vi "LVClass_CameraSet dtor.vi"(0 "CameraSet.lvclass":refnum<class "CameraSet.lvclass">, 11 "error in (no error)":errorcluster) -> (4 "CameraSet.lvclass":refnum<class "CameraSet.lvclass">, 15 "error out":errorcluster)   [LabVIEW 2020, in "CameraSet.lvclass"]
doc: "CameraSet destructor.\n\n--------------------------------------------------------------------------------\n\n<B>camera_setIn </B> : CameraSet object.\n<B>camera_setOut </B> : CameraSet object.\n<B>ErrorIn </B> : Error\n<B>ErrorOut </B> : Error\n\n--------------------------------------------------------------------------------"
uses:
  CameraSet.lvclass
  CameraSet.lvclass/CameraSet.ctl
  CameraSet.ctl
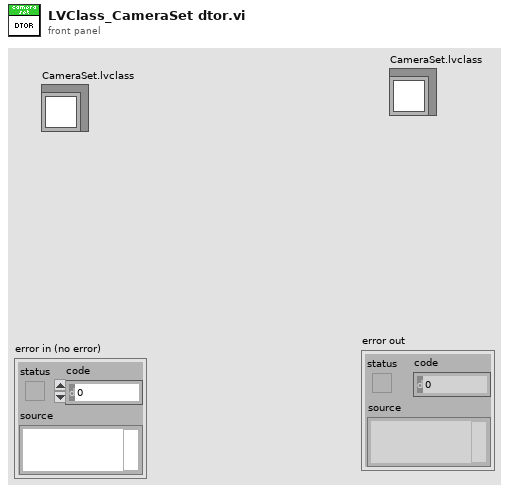
[diagram p1: front panel]
types:
  T1 = typedef "CameraSet.ctl" = i32
  T2 = typedef "Handle creation.ctl" = enum16{"By ctor", "By write function"}
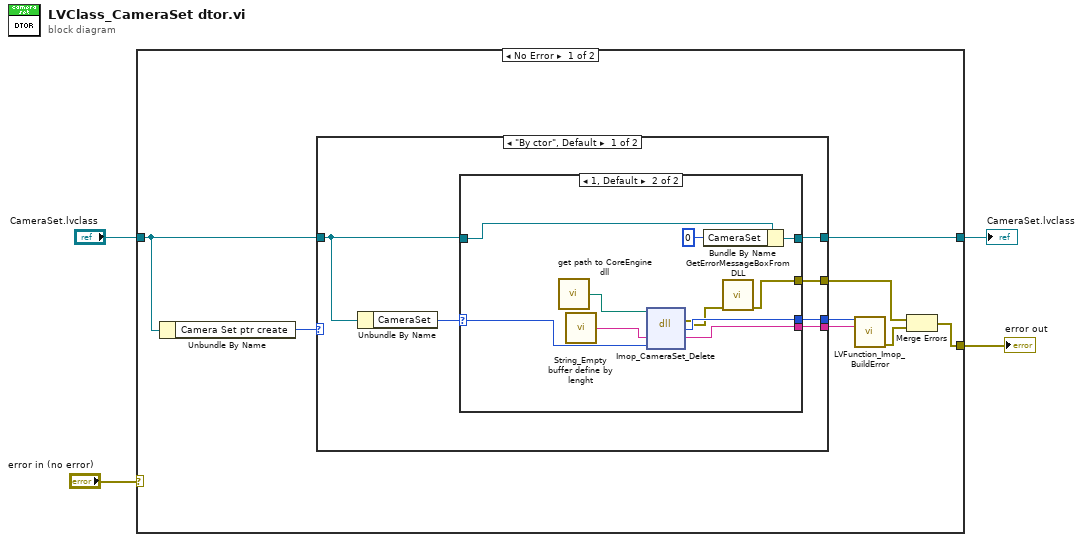
[diagram p0: block diagram]
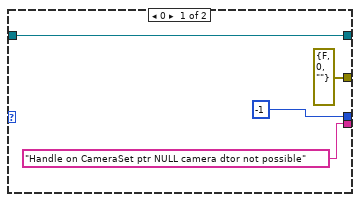
[diagram p2: hidden frame]
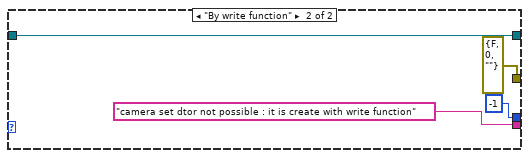
[diagram p3: hidden frame]
diagram:
  n1 = case shown="No Error" "error in (no error)" {
    selector: "error in (no error)" -> [_ w37]
    tunnel: "CameraSet.lvclass" -> [w9 w38]
    tunnel: [w10 w38] -> w2
    tunnel: [w5 w37] -> w1
    frame No Error {
      n2 = Unbundle By Name(w9) -> ("Camera Set ptr create"=w8:T2)
      n3 = case shown="\"By ctor\", Default" w8 {
        tunnel: [w18 "camera set dtor not possible : it is create with write function" ("message")] -> w12
        tunnel: [w17 -1] -> w11
        tunnel: [w16 w34] -> w10
        tunnel: w9 -> [w15 w34]
        tunnel: [w13 errorcluster {"status"=FALSE, "code"=0, "source"=""} ("error OUT")] -> w7
        frame "By ctor", Default {
          n4 = Unbundle By Name(w15) -> ("CameraSet"=w14:T1)
          n5 = case shown="1, Default" w14 {
            selector: w14 -> [_ w29]
            tunnel: ["Handle on CameraSet ptr NULL camera dtor not possible" ("message") w31] -> w18
            tunnel: [-1 w30] -> w17
            tunnel: w15 -> [w20 w26]
            tunnel: [w20 w25] -> w16
            tunnel: [errorcluster {"status"=FALSE, "code"=0, "source"=""} ("error OUT") w23] -> w13
            frame 0 {
            }
            frame 1, Default {
              n6 = call "get path to CoreEngine dll.vi"() -> ("path to c_interface_vc100.dll"=w28:path)  [unwired: 12 in, 3 out]
              n7 = call "String_Empty buffer define by lenght.vi"() -> ("Empty buffer"=w32:string)  [unwired: 1 in]
              n8 = dll-call lib="D:/soft/HASO_v3/SVN_trunk/ImOpCoreEngine4_LV2011/DLLs/c_interface_vc100.dll" fn="Imop_CameraSet_Delete"(path in=w28, "message"=w32, "objet"=w29) -> (error out=w27:errorcluster, "return type"=w30:i32, "message"=w31:string)  [unwired: 3 in, 1 out]
              n9 = Bundle By Name(cluster=w26, "CameraSet"=T1 0) -> (w25:refnum<class "CameraSet.lvclass">)
              n10 = call "GetErrorMessageBoxFromDLL.vi"("error IN"=w27) -> ("error OUT"=w23:errorcluster)  [unwired: 10 in]
            }
          }
        }
        frame "By write function" {
        }
      }
      n11 = call "LVFunction_Imop_BuildError.vi"("code"=w11, "String to Prepend to source (\"\")"=w12) -> ("error out"=w6:errorcluster)  [unwired: 13 in]
      n12 = Merge Errors(w7, w6) -> (w5:errorcluster)
    }
    frame Error {
    }
  }
  "CameraSet.lvclass" <- w2
  "error out" <- w1
